vi "Stop.vi"(8 "error in (no error)":errorcluster, 11 "Task in":refnum<class "DSP.lvclass">) -> (0 "error out":errorcluster, 3 "connection ID":i32)   [LabVIEW 2009, in "MicroDAQ.lvlib" / "DSP.lvclass"]
uses:
  <instrlib>/MicroDAQ/Channel/DSP/DSP.lvclass
  <instrlib>/MicroDAQ/Mlink library wraper/mlink.lvlib
  <instrlib>/MicroDAQ/Channel/Channel.lvclass
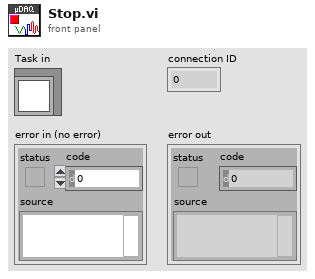
[diagram p1: front panel]
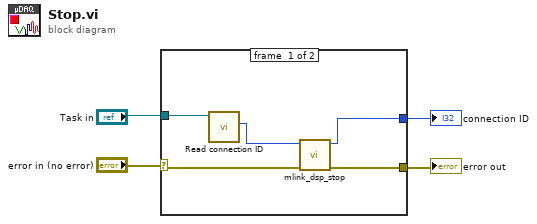
[diagram p0: block diagram]
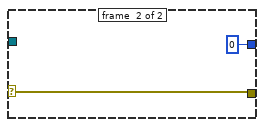
[diagram p2: hidden frame]
diagram:
  n1 = case shown="No Error" "error in (no error)" {
    selector: "error in (no error)" -> [w7 w11]
    tunnel: "Task in" -> [w9 _]
    tunnel: [w6 w11] -> w2
    tunnel: [w5 0 ("connection ID out")] -> w1
    frame #0 {
      n2 = call <instrlib>:"Read connection ID.vi"("Task in"=w9) -> ("connection ID"=w8:i32)  [unwired: 9 in, 1 out]
      n3 = call <instrlib>:"mlink_dsp_stop.vi"("error in (no error)"=w7, "connection ID"=w8) -> ("error out"=w6:errorcluster, "connection ID out"=w5:i32)  [unwired: 8 in]
    }
    frame #1 {
    }
  }
  "error out" <- w2
  "connection ID" <- w1
